vi "read_stream.vi"(7 "Acquisiton Config":T1 {"TC 2 Offset" format="%#_f"; "TC 2 Scale" format="%#_f"; "TC 1 Offset" format="%#_f"; "TC 1 Scale" format="%#_f"}, 8 "error in":errorcluster, 9 "NumReadAddresses":i32, 10 "ScansPerRead Out":i32, 11 "Handle In":i32) -> (0 "error out":errorcluster={"status"=TRUE, "code"=8605, "source"="LJM_eWriteAddresses.vi"}, 2 "Results":T2 {"CJTemp [K]" format="%#_f"; "TC Voltage [V]" format="%#_f"; "TC Temp. [degC]" format="%#_f"; "Current RMS [A]" format="%#_f"}, 3 "Handle Out":i32)   [LabVIEW 2025, in "LabJackEKG.lvlib"]
uses:
  LabJackEKG.lvlib
  Typedefs/ConnectionInfo.ctl
  Typedefs/ReadStreamData.ctl
  Typedefs/AcqusitionConfig.ctl
panel:
  in  "IP Address (LJM_idANY )":string="LJM_idANY"
  out "Connection Info":T3={"IPAddress"="192.168.1.8", "Port"=502, "DeviceType"=8, "ConnectionType"=3, "SerialNumber"=480010568, "MaxBytesPerPacket"=1040}
  in  "Initialize":bool
  out "Loop Time [ms]":dbl=0.008400000297115184 format="%.1f"
  in  "Period [ms]":i32=500 min=1 max=60000
  in  "Read Continuous":bool
  # "Driver Testing"
  # "LabJack V0.10\nRead Clamps / Stream"
  # "09.05.2025"
  # "Blaz Kelbl"
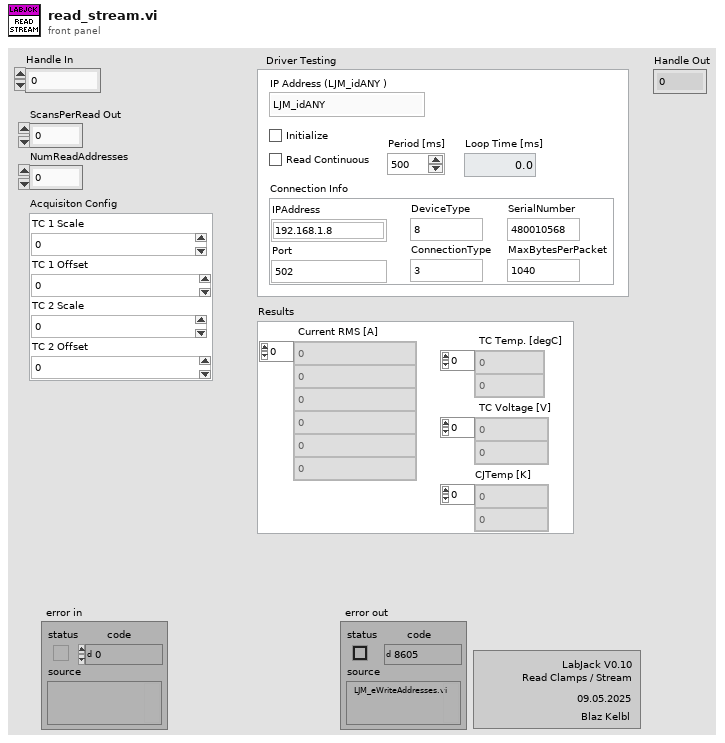
[diagram p1: front panel]
types:
  T1 = typedef "LabJackEKG.lvlib/AcqusitionConfig.ctl" = cluster{"TC 1 Scale":dbl, "TC 1 Offset":dbl, "TC 2 Scale":dbl, "TC 2 Offset":dbl}
  T2 = typedef "LabJackEKG.lvlib/ReadStreamData.ctl" = cluster{"Current RMS [A]":dbl[], "TC Temp. [degC]":dbl[], "TC Voltage [V]":dbl[], "CJTemp [K]":dbl[]}
  T3 = typedef "LabJackEKG.lvlib/ConnectionInfo.ctl" = cluster{"IPAddress":string, "Port":i32, "DeviceType":i32, "ConnectionType":i32, "SerialNumber":i32, "MaxBytesPerPacket":i32}
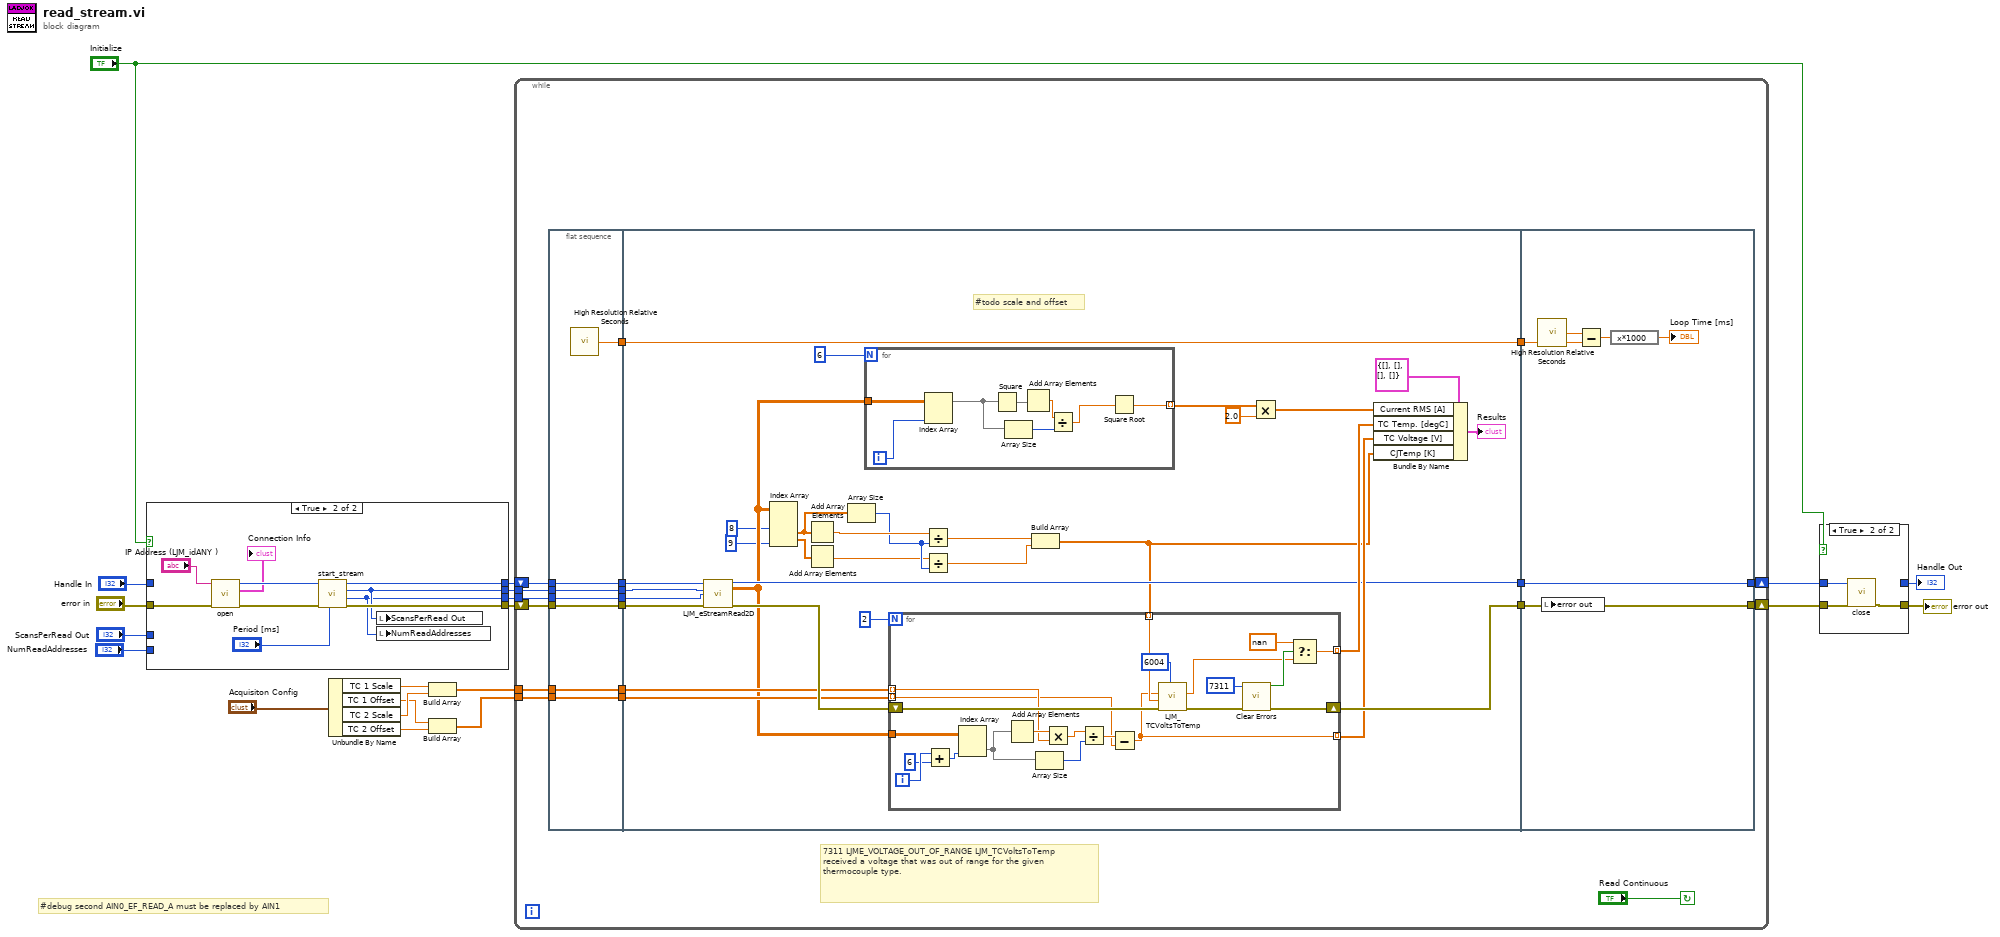
[diagram p0: block diagram]
diagram:
  # "#debug second AIN0_EF_READ_A must be replaced by AIN1"
  n1 = case shown="True" "Initialize" {
    tunnel: "error in" -> [w23 w34]
    tunnel: [w23 w30] -> w19
    tunnel: [w24 w29] -> w18
    tunnel: "Handle In" -> [w24 _]
    tunnel: [w21 w27] -> w10
    tunnel: [w22 w26] -> w11
    tunnel: "NumReadAddresses" -> [w22 _]
    tunnel: "ScansPerRead Out" -> [w21 _]
    frame False {
    }
    frame True {
      n2 = call "open.vi"("error in"=w34, "IP Address (LJM_idANY )"="IP Address (LJM_idANY )") -> ("error out"=w33:errorcluster, "Connection Info"=→"Connection Info":T3, "Handle"=w32:i32)  [unwired: 7 in]
      n3 = call "start_stream.vi"("Period [ms]"="Period [ms]", "error in (no error)"=w33, "Handle In"=w32) -> ("error out"=w30:errorcluster, "NumReadAddresses"=w26:i32, "ScansPerRead Out"=w27:i32, "Handle Out"=w29:i32)  [unwired: 5 in]
      n4 = local write "ScansPerRead Out"(w27) -> ()
      n5 = local write "NumReadAddresses"(w26) -> ()
    }
  }
  n6 = Unbundle By Name("Acquisiton Config") -> ("TC 1 Scale"=w7:dbl, "TC 1 Offset"=w5:dbl, "TC 2 Scale"=w6:dbl, "TC 2 Offset"=w4:dbl)
  n7 = Build Array(w7, w6) -> (w2:dbl[])
  n8 = Build Array(w5, w4) -> (w1:dbl[])
  n9 = while {
    shift-right: [w48] -> w12
    shift-left: w19 -> [w51]
    tunnel: w11 -> [w41]
    tunnel: w10 -> [w42]
    shift-right: [w52] -> w17
    shift-left: w18 -> [w53]
    tunnel: w2 -> [w38]
    tunnel: w1 -> [w36]
    stop <- "Read Continuous" continue-if-true
    # "7311\tLJME_VOLTAGE_OUT_OF_RANGE\tLJM_TCVoltsToTemp received a voltage that was out of range for the given thermocouple type."
    n10 = flat-sequence {
      tunnel: w51 -> [w59]
      tunnel: w53 -> [w60]
      tunnel: [w60] -> w45
      tunnel: [w59] -> w44
      tunnel: [w58] -> w43
      tunnel: w42 -> [w57]
      tunnel: w41 -> [w56]
      tunnel: [w57] -> w40
      tunnel: [w56] -> w39
      tunnel: w38 -> [w55]
      tunnel: [w55] -> w37
      tunnel: w36 -> [w54]
      tunnel: [w54] -> w35
      tunnel: [w72] -> w50
      tunnel: [w81] -> w49
      tunnel: w45 -> [w85]
      tunnel: w44 -> [w87]
      tunnel: [w90] -> w47
      tunnel: w43 -> [w90]
      tunnel: w40 -> [w84]
      tunnel: w39 -> [w83]
      tunnel: w37 -> [w74]
      tunnel: w35 -> [w73]
      tunnel: [w125] -> w48
      tunnel: [w126] -> w52
      tunnel: w50 -> [w126]
      tunnel: w49 -> [w125]
      tunnel: w47 -> [w122]
      frame #0 {
        n11 = call <vilib>:"High Resolution Relative Seconds.vi"() -> ("relative seconds"=w58:dbl)
      }
      frame #1 {
        # "#todo scale and offset"
        n12 = call <vilib>:"LJM_eStreamRead2D.vi"("Handle In"=w85, "ScansPerRead"=w84, "NumAddresses"=w83, "error in"=w87) -> ("Handle Out"=w72:i32, "aData Out"=w71:dbl[][], "error out"=w86:errorcluster)  [unwired: 7 in, 2 out]
        n13 = Index Array(array=w71, index (col) #1=8 ("disabled index (col)"), index (col) #2=9 ("index (col)")) -> (element #1=w69:dbl[], element #2=w66:dbl[])  [unwired: 2 in]
        n14 = Add Array Elements(numeric array=w69) -> (sum=w68:dbl)
        n15 = Add Array Elements(numeric array=w66) -> (sum=w64:dbl)
        n16 = Array Size(array=w69) -> (size(s)=w65:i32)
        n17 = for {
          N: 6 -> [_]
          tunnel: w71 -> [w120]
          tunnel: [w114] -> w89 mode=indexing
          i -> [w113]
          n18 = Index Array(array=w120, index (col)=w113) -> (element=w118:dbl[])  [unwired: 1 in]
          n19 = Square(x=w118) -> (x^2=w115:dbl[])
          n20 = Array Size(array=w118) -> (size(s)=w117:i32)
          n21 = Add Array Elements(numeric array=w115) -> (sum=w116:dbl)
          n22 = Divide(x=w116, y=w117) -> (x/y=w119:dbl)
          n23 = Square Root(x=w119) -> (sqrt(x)=w114:dbl)
        }
        n24 = Divide(x=w68, y=w65) -> (x/y=w62:dbl)
        n25 = Divide(x=w64, y=w65) -> (x/y=w63:dbl)
        n26 = Build Array(w62, w63) -> (w61:dbl[])
        n27 = for {
          N: 2 -> [_]
          tunnel: w71 -> [w112]
          shift-right: [w98] -> w81
          shift-left: w86 -> [w105]
          tunnel: [w96] -> w77 mode=indexing
          tunnel: [w100] -> w76 mode=indexing
          tunnel: w61 -> [w103] mode=indexing
          tunnel: w74 -> [w101] mode=indexing
          tunnel: w73 -> [w99] mode=indexing
          i -> [w111]
          n28 = Add(x=w111, y=6) -> (x+y=w92:i32)
          n29 = Index Array(array=w112, index (col)=w92) -> (element=w108:dbl[])  [unwired: 1 in]
          n30 = Add Array Elements(numeric array=w108) -> (sum=w109:dbl)
          n31 = Array Size(array=w108) -> (size(s)=w110:i32)
          n32 = Multiply(x=w109, y=w101) -> (x*y=w102:dbl)
          n33 = Divide(x=w102, y=w110) -> (x/y=w104:dbl)
          n34 = Subtract(x=w104, y=w99) -> (x-y=w100:dbl)
          n35 = call <vilib>:"LJM_TCVoltsToTemp.vi"("TCType"=6004, "error in"=w105, "CJTempK"=w103, "TCVolts"=w100) -> ("error out"=w106:errorcluster, "TCTempC"=w93:dbl)  [unwired: 4 in, 2 out]
          n36 = call <vilib>:"Clear Errors.vi"("error in (no error)"=w106, "specific error code to clear (0: all)"=7311) -> ("error out"=w98:errorcluster, "specific error cleared?"=w95:bool)  [unwired: 4 in]
          n37 = Select(t=nan, s=w95, f=w93) -> (s? t:f=w96:dbl)
        }
        n38 = Multiply(x=w89, y=2.0 ("x")) -> (x*y=w79:dbl[])
        n39 = Bundle By Name(cluster=T2 {"Current RMS [A]"=[], "TC Temp. [degC]"=[], "TC Voltage [V]"=[], "CJTemp [K]"=[]} ("Results"), "Current RMS [A]"=w79, "TC Temp. [degC]"=w77, "TC Voltage [V]"=w76, "CJTemp [K]"=w61) -> (→"Results":T2)
      }
      frame #2 {
        n40 = call <vilib>:"High Resolution Relative Seconds.vi"() -> ("relative seconds"=w124:dbl)
        n41 = local write "error out"(w125) -> ()
        n42 = Subtract(x=w124, y=w122) -> (x-y=w123:dbl)
        n43 = expression code="x*1000"(w123) -> (→"Loop Time [ms]":dbl)
      }
    }
  }
  n44 = case shown="True" "Initialize" {
    tunnel: w17 -> [w128 w129]
    tunnel: w12 -> [w127 w130]
    tunnel: [w128 _] -> w13
    tunnel: [w127 w131] -> w16
    frame False {
    }
    frame True {
      n45 = call "close.vi"("error in"=w130, "Handle"=w129) -> ("error out"=w131:errorcluster)  [unwired: 9 in]
    }
  }
  "error out" <- w16
  "Handle Out" <- w13
